vi "Read function key.vi"(8 "error in (no error)":errorcluster, 10 "function key":u16(ring)=1 items=["F1"=1, "F2"=2], 11 "connection ID in":i32=-1) -> (0 "error out":errorcluster, 2 "state":bool, 3 "connection ID out":i32)   [LabVIEW 2009, in "MicroDAQ.lvlib"]
doc: "This function reads F1/F2 function key state."
uses:
  <instrlib>/MicroDAQ/MicroDAQ.lvlib
  <instrlib>/MicroDAQ/Mlink library wraper/mlink.lvlib
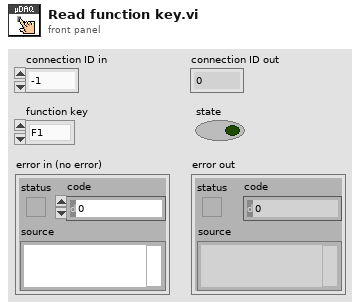
[diagram p1: front panel]
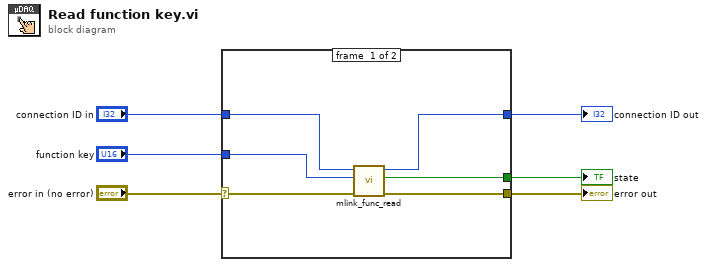
[diagram p0: block diagram]
diagram:
  n1 = case shown="No Error" "error in (no error)" {
    selector: "error in (no error)" -> [w10 w13]
    tunnel: "function key" -> [w12 _]
    tunnel: "connection ID in" -> [w11 w14]
    tunnel: [w9 w14] -> w3
    tunnel: [w8 _] -> w2
    tunnel: [w7 w13] -> w1
    frame #0 {
      n2 = call <instrlib>:"mlink_func_read.vi"("error in (no error)"=w10, "function key"=w12, "connection ID"=w11) -> ("error out"=w7:errorcluster, "state"=w8:bool, "link_fd out"=w9:i32)  [unwired: 6 in]
    }
    frame #1 {
    }
  }
  "connection ID out" <- w3
  "state" <- w2
  "error out" <- w1
